vi "Text2EEPROM.vi"(10 "dimension size":i32=27, 11 "EEPROM Data":string) -> (3 "EEPROM data":u8[][](array[numeric]) format="%02x")   [LabVIEW 2015]
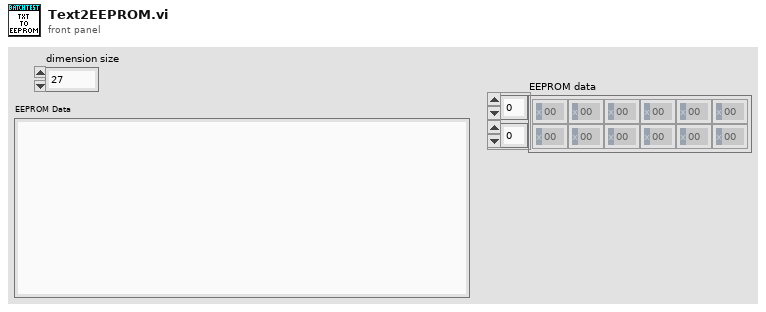
[diagram p1: front panel]
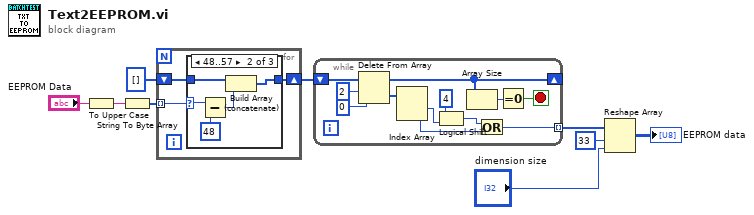
[diagram p0: block diagram]
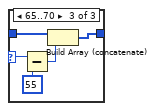
[diagram p3: hidden frame]
diagram:
  n1 = To Upper Case(1:"EEPROM Data") -> (0:w9:string)
  n2 = String To Byte Array(string=w9) -> (unsigned byte array=w7:u8[])
  n3 = for {
    tunnel: w7 -> [w12] mode=indexing
    shift-right: [w11] -> w3
    shift-left: u8[] [] ("EEPROM data") -> [w10]
    n4 = case shown="48..57" w12 {
      selector: w12 -> [_ w17 w22]
      tunnel: [w13 w15 w20] -> w11
      tunnel: w10 -> [w13 w18 w23]
      frame Default {
      }
      frame 48..57 {
        n5 = Subtract(x=w17, y=u8 48) -> (x-y=w14:u8)
        n6 = Build Array (concatenate)(w18, w14) -> (w15:u8[])
      }
      frame 65..70 {
        n7 = Subtract(x=w22, y=u8 55) -> (x-y=w19:u8)
        n8 = Build Array (concatenate)(w23, w19) -> (w20:u8[])
      }
    }
  }
  n9 = while {
    shift-right: [w27] -> _
    shift-left: w3 -> [w35]
    tunnel: [w28] -> w2 mode=indexing
    stop <- w25 stop-if-true
    n10 = Delete From Array(array=w35, length=2, index=0) -> (deleted portion=w33:u8[], array with subset deleted=w27:u8[])
    n11 = Index Array(array=w33) -> (element #1=w31:u8, element #2=w29:u8)  [unwired: 2 in]
    n12 = Logical Shift(y=i8 4, x=w31) -> (x << y=w30:u8)
    n13 = Array Size(array=w27) -> (size(s)=w26:i32)
    n14 = Or(x=w30, y=w29) -> (x .or. y?=w28:u8)
    n15 = Equal To 0?(x=w26) -> (x = 0?=w25:bool)
  }
  n16 = Reshape Array(w2, 33 ("dimension size"), "dimension size") -> (→"EEPROM data":u8[][])
